vi "XIPIN_Virtex-7_FPGA_Gen3_Integrated_Block_for_PCI_Express_4_1.vi"   [LabVIEW 2017]
doc: "The Xilinx 7 Series Gen3 Integrated Block for PCI Express (1-lane, 2-lane, 4-lane, and 8-lane) in conjunction with flexible 7-Series architectural features such as integrated GTs (Gigabit Transceivers) and BRAM (Block RAMs) are used to implement a PCI Express Base Specification v3.0 compliant PCI Express Endpoint.\n------------------------------------\n<b>Need License</b> : No\n<b>Interface</b> : AXI4-Stream"
uses:
  <vilib>/rvi/XilinxIP/XIPIN_XNode/niFpgaXIPIN.xnode
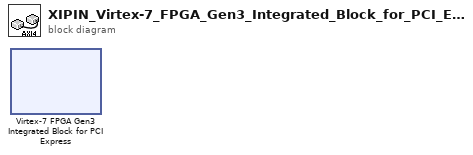
[diagram p0: block diagram]
diagram:
  n1 = xnode ("Virtex-7 FPGA Gen3 Integrated Block for PCI Express")() -> ()
